vi "定时启动 (子VI).vi"   [LabVIEW 2016, in "斯坦道CODMn.lvlib"]
types:
  T1 = enum16{"启动测量", "标样核查", "零点核查", "跨度核查", "空白测试", "平行样测试", "加标回收", "空白校准", "标样校准", "初始化（清洗）", "停止测试", "仪器重启", "校时", "模式设置", "测量间隔设置"}
  T2 = cluster{"测量模式":enum16{"水样测量", "标样核查", "零点核查", "跨度核查", "空白测试", "加标回收", "平行样", "校零", "校标"}}
  T3 = cluster{"控制命令":enum16{"启动测量", "标样核查", "零点核查", "跨度核查", "空白测试", "平行样测试", "加标回收", "空白校准", "标样校准", "初始化（清洗）", "停止测试", "仪器重启", "校时", "模式设置", "测量间隔设置"}, "周期设置类型":enum16{"定点启动", "间隔启动"}, "定时功能启用":bool, "定时间隔":dbl, "24H周期设置":bool[], "零点核查时间":u16, "跨度核查时间":u16, "质控频次":enum16{"关闭", "每天", "星期一", "星期二", "星期三", "星期四", "星期五", "星期六", "星期日"}}
  T4 = enum16{"关闭", "每天", "星期一", "星期二", "星期三", "星期四", "星期五", "星期六", "星期日"}
  T5 = typedef "LVDateTimeRec.ctl" = cluster{"秒数的小数部分":dbl, "秒":i32, "分":i32, "时":i32, "日":i32, "月":i32, "年":i32, "天数（周）":i32, "天数（年）":i32, "DST":i32}
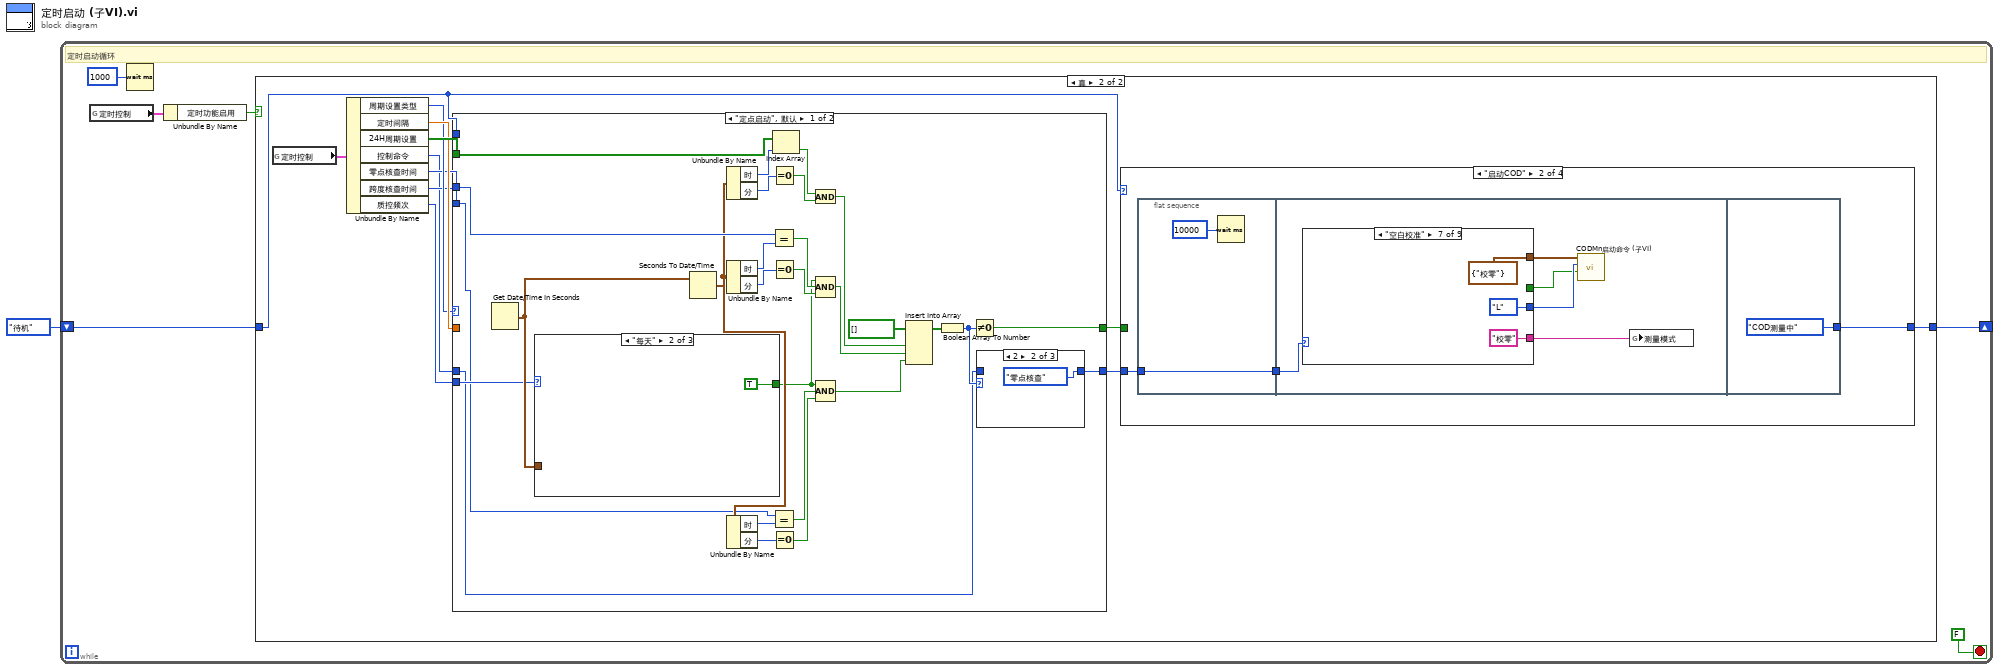
[diagram p0: block diagram]
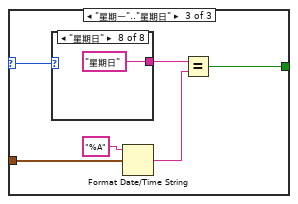
[diagram p4: hidden frame]
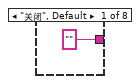
[diagram p5: hidden frame]
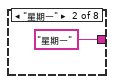
[diagram p6: hidden frame]
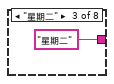
[diagram p7: hidden frame]
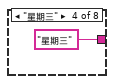
[diagram p8: hidden frame]
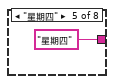
[diagram p9: hidden frame]
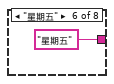
[diagram p10: hidden frame]
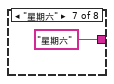
[diagram p11: hidden frame]
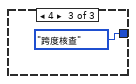
[diagram p13: hidden frame]
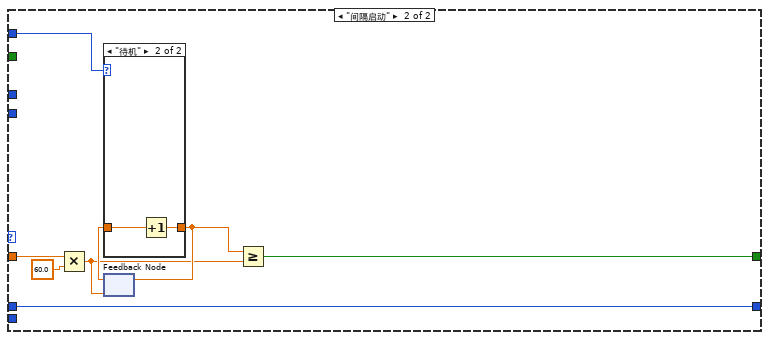
[diagram p14: hidden frame]
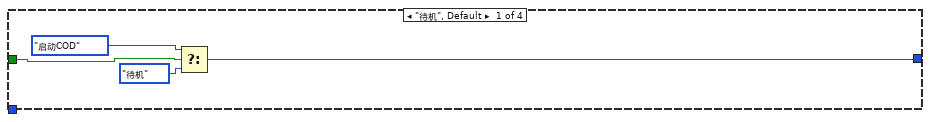
[diagram p16: hidden frame]
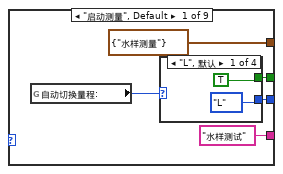
[diagram p17: hidden frame]
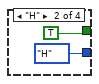
[diagram p18: hidden frame]
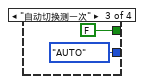
[diagram p19: hidden frame]
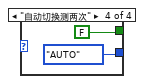
[diagram p20: hidden frame]
diagram:
  n1 = while {
    shift-right: [w6] -> _
    shift-left: enum16{"待机", "启动COD", "COD测量中", "延时"}."待机" -> [w5]
    stop <- FALSE stop-if-true
    # "定时启动循环"
    n2 = global read "CODMn断电保存全局变量.vi" "定时控制"() -> (w4:T3)
    n3 = Wait (ms)(milliseconds to wait=u32 1000 ("等待时间（毫秒）")) -> ()  [unwired: 1 out]
    n4 = Unbundle By Name(w4) -> ("定时功能启用"=w3:bool)
    n5 = case shown="真" w3 {
      tunnel: [w8 w20] -> w6
      tunnel: w5 -> [w8 w19]
      frame False {
      }
      frame True {
        n6 = global read "CODMn断电保存全局变量.vi" "定时控制"() -> (w13:T3)
        n7 = Unbundle By Name(w13) -> ("周期设置类型"=w14:enum16{"定点启动", "间隔启动"}, "定时间隔"=w15:dbl, "24H周期设置"=w16:bool[], "控制命令"=w9:T1, "零点核查时间"=w12:u16, "跨度核查时间"=w10:u16, "质控频次"=w11:T4)
        n8 = case shown="\"定点启动\", 默认" w14 {
          tunnel: w15 -> [_ w71]
          tunnel: w16 -> [w48 _]
          tunnel: w19 -> [_ w74]
          tunnel: [w24 w69] -> w18
          tunnel: w12 -> [w47 _]
          tunnel: w11 -> [w25 _]
          tunnel: w10 -> [w23 _]
          tunnel: w9 -> [w22 w67]
          tunnel: [w21 w67] -> w17
          frame "定点启动", Default {
            n9 = Get Date/Time In Seconds() -> (seconds since 1Jan1904=w43:timestamp)
            n10 = case shown="\"每天\"" w25 {
              selector: w25 -> [_ _ w53]
              tunnel: w43 -> [_ _ w54]
              tunnel: [_ TRUE w50] -> w32
              frame "关闭", Default {
              }
              frame "每天" {
              }
              frame "星期一".."星期日" {
                n11 = case shown="\"星期日\"" w53 {
                  tunnel: ["" ("时间格式字符串(%c)") "星期一" ("时间格式字符串(%c)") "星期二" ("时间格式字符串(%c)") "星期三" ("时间格式字符串(%c)") "星期四" ("时间格式字符串(%c)") "星期五" ("时间格式字符串(%c)") "星期六" ("时间格式字符串(%c)") "星期日" ("时间格式字符串(%c)")] -> w52
                  frame "关闭", Default {
                  }
                  frame "星期一" {
                  }
                  frame "星期二" {
                  }
                  frame "星期三" {
                  }
                  frame "星期四" {
                  }
                  frame "星期五" {
                  }
                  frame "星期六" {
                  }
                  frame "星期日" {
                  }
                }
                n12 = Format Date/Time String(time format string (%c)="%A" ("时间格式字符串(%c)"), seconds (now)=w54) -> (date/time string=w51:string)  [unwired: 1 in]
                n13 = Equal?(x=w52, y=w51) -> (x = y?=w50:bool)
              }
            }
            n14 = Seconds To Date/Time(time stamp (now)=w43) -> (date time rec=w33:T5)  [unwired: 1 in]
            n15 = Unbundle By Name(w33) -> ("时"=w46:i32, "分"=w45:i32)
            n16 = Unbundle By Name(w33) -> ("时"=w40:i32, "分"=w41:i32)
            n17 = Unbundle By Name(w33) -> ("时"=w35:i32, "分"=w34:i32)
            n18 = Equal?(x=w47, y=w40) -> (x = y?=w39:bool)
            n19 = Equal?(x=w23, y=w35) -> (x = y?=w36:bool)
            n20 = Equal To 0?(x=w45) -> (x = 0?=w44:bool)
            n21 = Equal To 0?(x=w41) -> (x = 0?=w38:bool)
            n22 = Equal To 0?(x=w34) -> (x = 0?=w37:bool)
            n23 = Index Array(array=w48, index=w46) -> (element=w42:bool)
            n24 = Compound Arithmetic op=AND ("复合运算")(w42, w44) -> (w30:bool)
            n25 = Compound Arithmetic op=AND ("复合运算")(w32, w39, w38) -> (w29:bool)
            n26 = Compound Arithmetic op=AND ("复合运算")(w32, w36, w37) -> (w28:bool)
            n27 = Insert Into Array(array=bool[] [], new element #1=w30, new element #2=w29, new element #3=w28) -> (w27:bool[])  [unwired: 1 in]
            n28 = Boolean Array To Number(Boolean array=w27) -> (number=w26:u32)
            n29 = Not Equal To 0?(x=w26) -> (x != 0?=w24:bool)
            n30 = case shown="2" w26 {
              tunnel: [w64 T1."零点核查" ("控制命令") T1."跨度核查" ("控制命令")] -> w21
              tunnel: w22 -> [w64 _ _]
              frame 0, Default {
              }
              frame 2 {
              }
              frame 4 {
              }
            }
          }
          frame "间隔启动" {
            n31 = Multiply(x=w71, y=60.0) -> (x*y=w68:dbl)
            n32 = feedback #1(w68) -> (w73:dbl)
            n33 = case shown="\"待机\"" w74 {
              tunnel: w73 -> [_ w76]
              tunnel: [_ w75] -> w72
              frame Default {
              }
              frame "待机" {
                n34 = Increment(x=w76) -> (x+1=w75:dbl)
              }
            }
            n35 = feedback-in #1(w72) -> ()
            n36 = Greater Or Equal?(x=w72, y=w68) -> (x >= y?=w69:bool)
          }
        }
        n37 = case shown="\"启动COD\"" w19 {
          tunnel: [w77 w83 w130 enum16{"待机", "启动COD", "COD测量中", "延时"}."待机"] -> w20
          tunnel: w18 -> [w80 _ _ _]
          tunnel: w17 -> [_ w81 _ _]
          frame "待机", Default {
            n38 = Select(t=enum16{"待机", "启动COD", "COD测量中", "延时"}."启动COD", s=w80, f=enum16{"待机", "启动COD", "COD测量中", "延时"}."待机") -> (s? t:f=w77:enum16{"待机", "启动COD", "COD测量中", "延时"})
          }
          frame "启动COD" {
            n39 = flat-sequence {
              tunnel: w81 -> [w85]
              tunnel: [w85] -> w82
              tunnel: w82 -> [w90]
              tunnel: [enum16{"待机", "启动COD", "COD测量中", "延时"}."COD测量中"] -> w83
              frame #0 {
                n40 = Wait (ms)(milliseconds to wait=u32 10000 ("等待时间（毫秒）")) -> ()  [unwired: 1 out]
              }
              frame #1 {
                n41 = case shown="\"空白校准\"" w90 {
                  tunnel: [T2 {"测量模式"=enum."水样测量"} ("启动测量模式") T2 {"测量模式"=enum."标样核查"} ("启动测量模式") T2 {"测量模式"=enum."空白测试"} ("启动测量模式") T2 {"测量模式"=enum."跨度核查"} ("启动测量模式") T2 {"测量模式"=enum."加标回收"} ("启动测量模式") T2 {"测量模式"=enum."平行样"} ("启动测量模式") T2 {"测量模式"=enum."校零"} ("启动测量模式") T2 {"测量模式"=enum."校标"} ("启动测量模式") T2 {"测量模式"=enum."零点核查"} ("启动测量模式")] -> w89
                  tunnel: ["水样测试" ("测量模式") "标样核查" ("测量模式") "空白测试" ("测量模式") "跨度核查" ("测量模式") "加标回收" ("测量模式") "平行样" ("测量模式") "校零" ("测量模式") "校标" ("测量模式") "零点核查" ("测量模式")] -> w88
                  tunnel: [w93 w104 enum32{"H", "L", "AUTO"}."L" ("CODMn跨度量程选择") w110 enum32{"H", "L", "AUTO"}."AUTO" ("CODMn跨度量程选择") enum32{"H", "L", "AUTO"}."AUTO" ("CODMn跨度量程选择") enum32{"H", "L", "AUTO"}."L" ("CODMn跨度量程选择") enum32{"H", "L", "AUTO"}."AUTO" ("CODMn跨度量程选择") w125] -> w87
                  tunnel: [w92 _ _ _ _ _ _ _ _] -> w86
                  frame "启动测量", Default {
                    n42 = global read "CODMn断电保存全局变量.vi" "自动切换量程:"() -> (w91:enum16{"L", "H", "自动切换测一次", "自动切换测两次"})
                    n43 = case shown="\"L\", 默认" w91 {
                      tunnel: [enum32{"H", "L", "AUTO"}."L" ("CODMn跨度量程选择") enum32{"H", "L", "AUTO"}."H" ("CODMn跨度量程选择") enum32{"H", "L", "AUTO"}."AUTO" ("CODMn跨度量程选择") enum32{"H", "L", "AUTO"}."AUTO" ("CODMn跨度量程选择")] -> w93
                      tunnel: [TRUE TRUE FALSE FALSE] -> w92
                      frame "L", Default {
                      }
                      frame "H" {
                      }
                      frame "自动切换测一次" {
                      }
                      frame "自动切换测两次" {
                      }
                    }
                  }
                  frame "标样核查" {
                    n44 = global read "CODMn断电保存全局变量.vi" "标样核查量程选择"() -> (w104:enum32{"H", "L", "AUTO"})
                  }
                  frame "空白测试" {
                  }
                  frame "跨度核查" {
                    n45 = global read "CODMn断电保存全局变量.vi" "CODMn跨度量程选择"() -> (w110:enum32{"H", "L", "AUTO"})
                  }
                  frame "加标回收" {
                  }
                  frame "平行样测试" {
                  }
                  frame "空白校准" {
                  }
                  frame "标样校准" {
                  }
                  frame "零点核查" {
                    n46 = global read "CODMn断电保存全局变量.vi" "零点核查量程选择"() -> (w125:enum32{"H", "L", "AUTO"})
                  }
                }
                n47 = call "CODMn启动命令 (子VI).vi"("强制切换"=w86, "CODMn量程切换"=w87, "启动测量模式"=w89) -> ()  [unwired: 9 in]
                n48 = global write "COD测量模式全局.vi" "测量模式"(w88) -> ()
              }
              frame #2 {
              }
            }
          }
          frame "COD测量中" {
            n49 = flat-sequence {
              tunnel: [w131] -> w129
              tunnel: [w138] -> w130
              tunnel: w129 -> [w138]
              frame #0 {
                n50 = global read "运行时序全局变量.vi" "多列列表框"() -> (w136:i32)
                n51 = Equal?(x=w136, y=0) -> (x = y?=w134:bool)
                n52 = Select(t=enum16{"待机", "启动COD", "COD测量中", "延时"}."延时", s=w134, f=enum16{"待机", "启动COD", "COD测量中", "延时"}."COD测量中") -> (s? t:f=w131:enum16{"待机", "启动COD", "COD测量中", "延时"})
              }
              frame #1 {
                n53 = Wait (ms)(milliseconds to wait=u32 5000 ("等待时间（毫秒）")) -> ()  [unwired: 1 out]
              }
            }
          }
          frame "延时" {
          }
        }
      }
    }
  }
